vi "tcp_comms.vi"() -> ()   [LabVIEW 2021]
panel:
  out "bytes written":i32
  out "Received Value 2":dbl
  out "Received Value 1":dbl
  out "String that is Received":string
  out "String that is Sent":string
  in  "SendValue2":dbl
  in  "Send Value1":dbl
  in  "stop":bool
  in  "SEND Button":bool
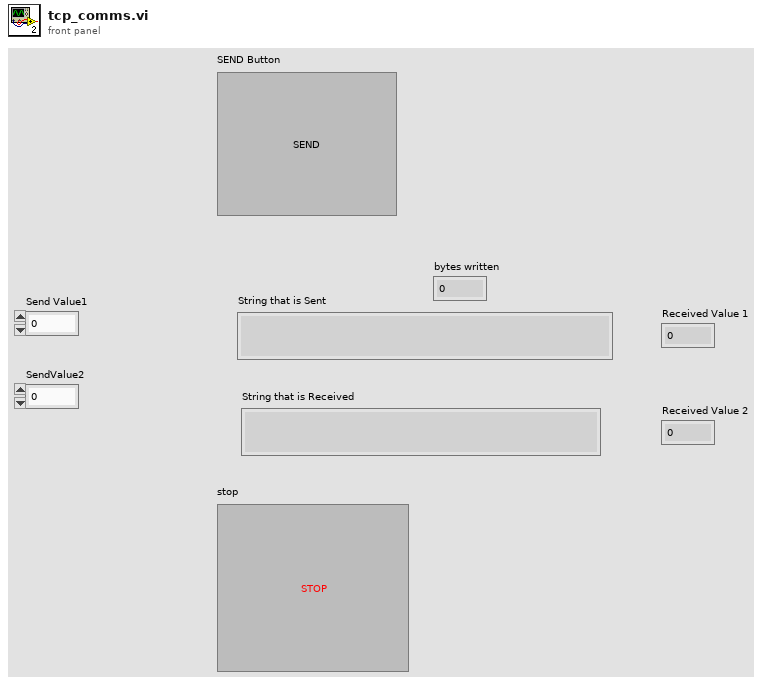
[diagram p1: front panel]
types:
  T1 = enum16{"Standard", "Buffered", "CRLF", "Immediate"}
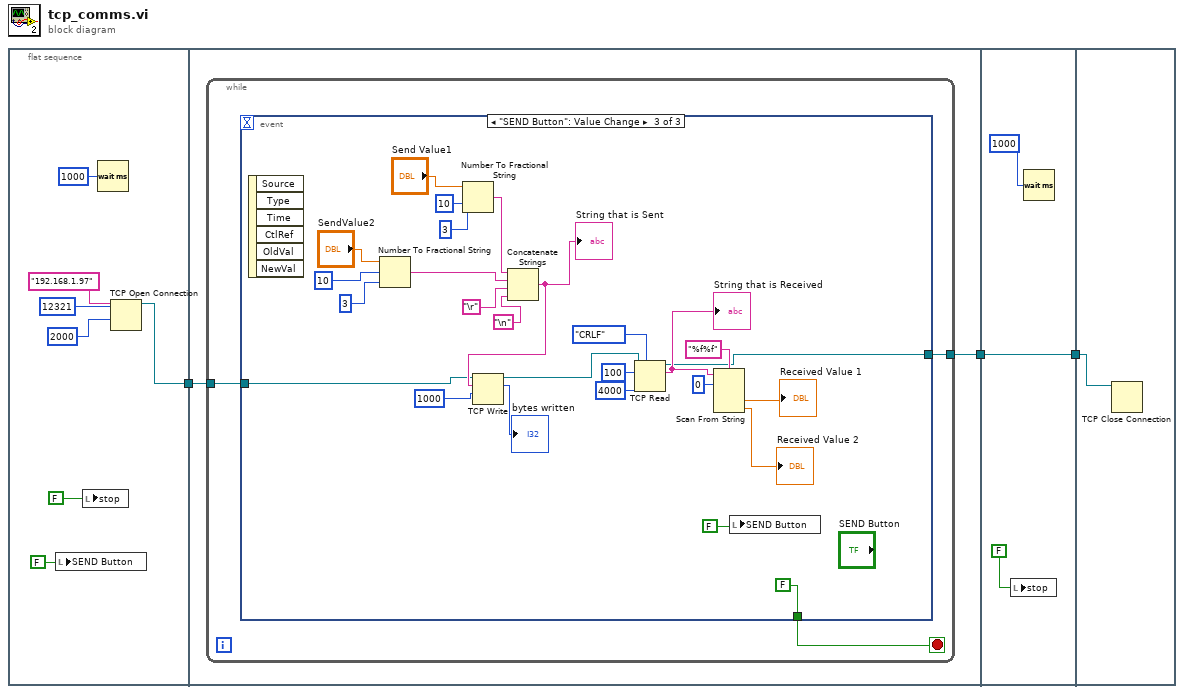
[diagram p0: block diagram]
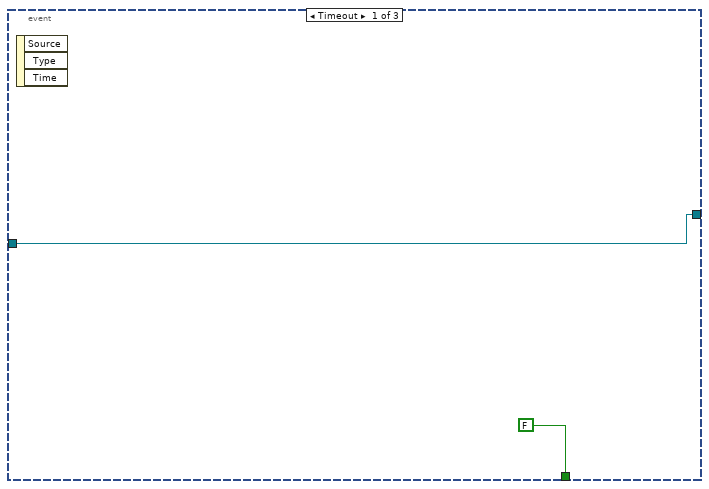
[diagram p2: hidden frame]
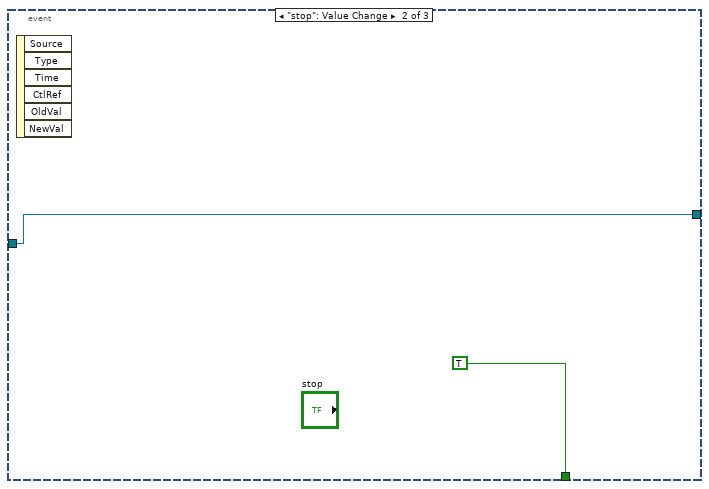
[diagram p3: hidden frame]
diagram:
  n1 = flat-sequence {
    tunnel: [w4] -> w1
    tunnel: [w12] -> w3
    tunnel: w1 -> [w11]
    tunnel: w3 -> [w47]
    tunnel: [w47] -> w2
    tunnel: w2 -> [w49]
    frame #0 {
      n2 = local write "SEND Button"(FALSE) -> ()
      n3 = local write "stop"(FALSE) -> ()
      n4 = Wait (ms)(milliseconds to wait=u32 1000) -> ()  [unwired: 1 out]
      n5 = TCP Open Connection(address="192.168.1.97", remote port or service name=u16 12321, timeout ms (60000)=2000) -> (connection ID=w4:refnum<k5>)  [unwired: 2 in, 1 out]
    }
    frame #1 {
      n6 = while {
        tunnel: [w14] -> w12
        tunnel: w11 -> [w13]
        stop <- w15 stop-if-true
        n7 = event shown="[2] \"SEND Button\": Value Change" {
          selector: _ -> [_ _ _]
          dyn-events: _ -> [_ _ _]
          timeout: _ -> [_ _ _]
          tunnel: w13 -> [w17 w18 w21]
          tunnel: [FALSE TRUE FALSE] -> w15
          tunnel: [w17 w18 w24] -> w14
          event Timeout {
            n8 = event-data() -> ()  [unwired: 1 in, 3 out]
          }
          event "stop": Value Change {
            n9 = event-data() -> ()  [unwired: 1 in, 6 out]
          }
          event "SEND Button": Value Change {
            n10 = event-data() -> ()  [unwired: 1 in, 6 out]
            n11 = Number To Fractional String(number="SendValue2", width (-)=i16 10, precision (6)=i16 3) -> (F-format string=w38:string)  [unwired: 1 in]
            n12 = Number To Fractional String(number="Send Value1", width (-)=i16 10, precision (6)=i16 3) -> (F-format string=w39:string)  [unwired: 1 in]
            n13 = Concatenate Strings(w39, w38, "\r", "\n") -> (w35:string)
            "String that is Sent" <- w35
            n14 = TCP Write(connection ID=w21, data in=w35, 9:1000 ("timeout ms (25000)")) -> (connection ID out=w20:refnum<k5>, bytes written=→"bytes written":i32)  [unwired: 1 in, 1 out]
            n15 = TCP Read(connection ID=w20, bytes to read=100, 7:T1."CRLF" ("mode (standard)"), 9:4000 ("timeout ms (25000)")) -> (connection ID out=w24:refnum<k5>, data out=w27:string)  [unwired: 1 in, 1 out]
            "String that is Received" <- w27
            n16 = Scan From String(format string="%f%f", input string=w27, initial scan location=u32 0) -> (output 1=→"Received Value 1":dbl, output 2=→"Received Value 2":dbl)  [unwired: 3 in, 3 out]
            n17 = local write "SEND Button"(FALSE) -> ()
          }
        }
      }
    }
    frame #2 {
      n18 = local write "stop"(FALSE) -> ()
      n19 = Wait (ms)(milliseconds to wait=u32 1000) -> ()  [unwired: 1 out]
    }
    frame #3 {
      n20 = TCP Close Connection(connection ID=w49) -> ()  [unwired: 2 in, 2 out]
    }
  }
